vi "acquireWhenClick.vi"() -> ()   [LabVIEW 2016]
uses:
  <vilib>/Utility/file.llb/Write Delimited Spreadsheet (DBL).vi
panel:
  out "即将记录":dbl=1.0
  out "osc stoped":bool
  in  "OSC in":refnum<visa-resource-name>
  in  "start":bool
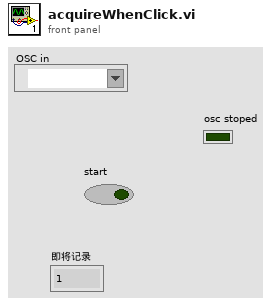
[diagram p1: front panel]
types:
  T1 = typedef "NI_Matrix.lvlib/RealMatrix.ctl" = dbl[][]
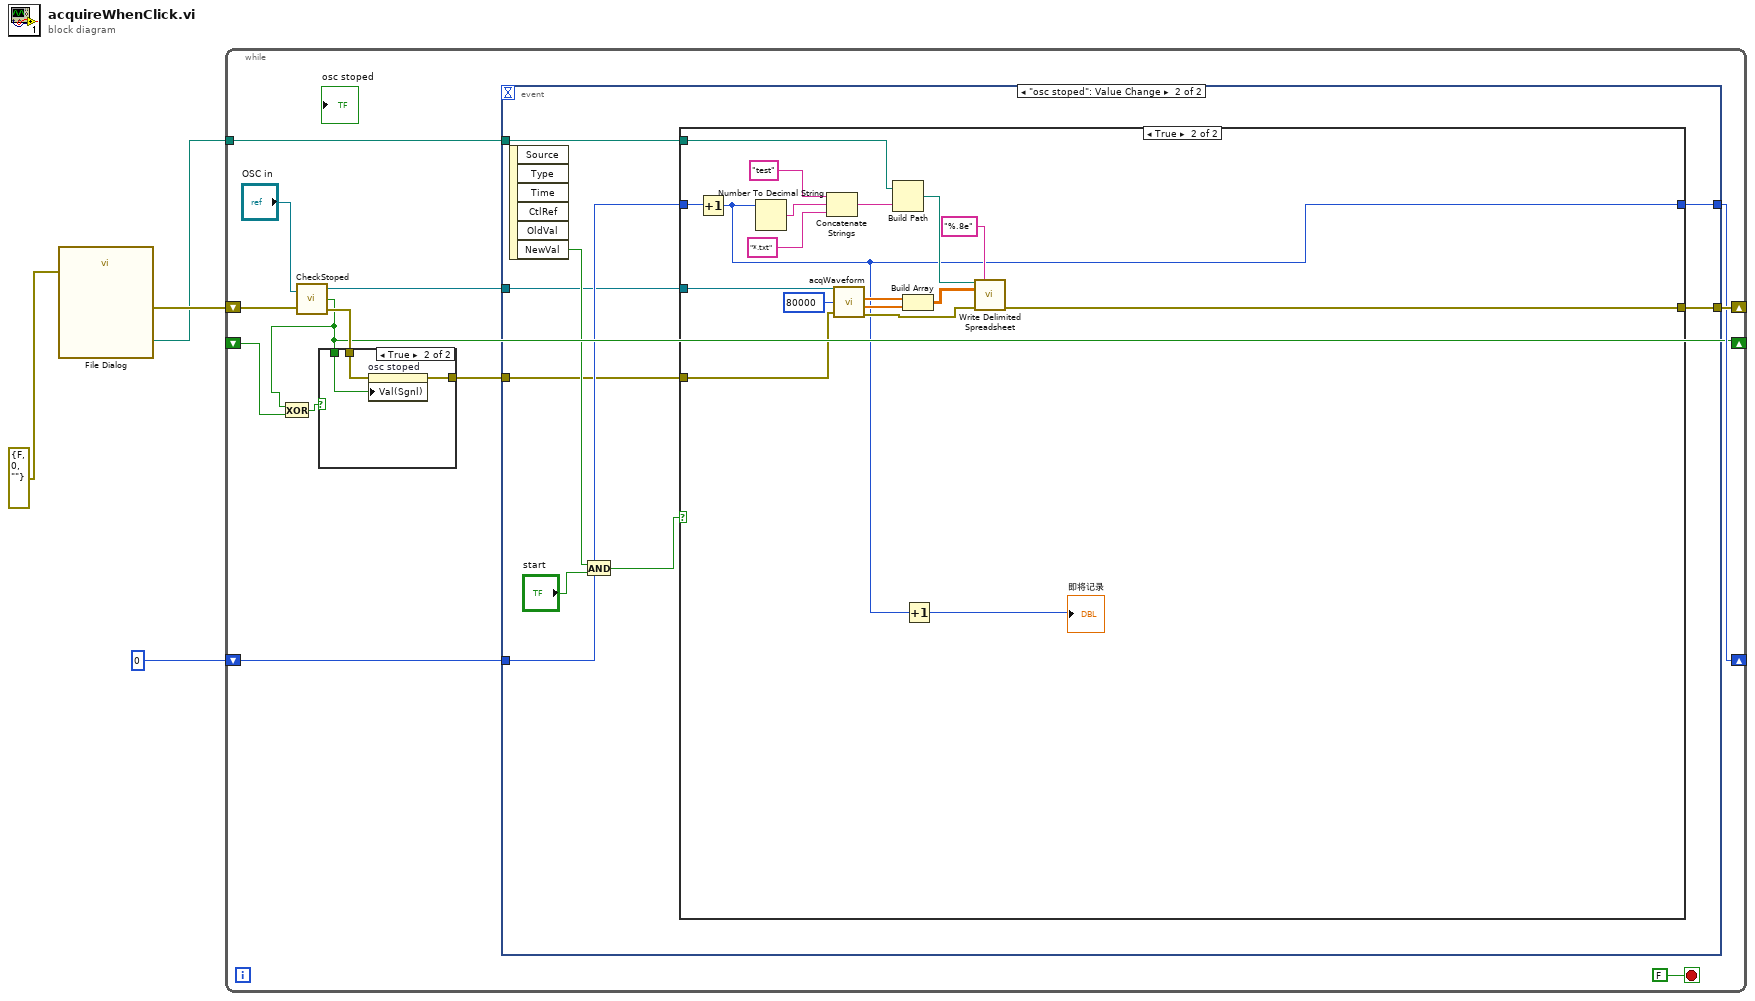
[diagram p0: block diagram]
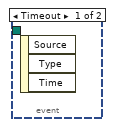
[diagram p3: hidden frame]
diagram:
  n1 = call "File Dialog"("error in"=errorcluster {"status"=FALSE, "code"=0, "source"=""} ("error in (no error)")) -> ("selected path"=w1:path, "error out"=w2:errorcluster)  [unwired: 11 in, 2 out]
  n2 = while {
    tunnel: w1 -> [w10]
    shift-right: [w9] -> _
    shift-left: w2 -> [w16]
    shift-right: [w8] -> _
    shift-left: 0 -> [w13]
    shift-right: [w6] -> _
    shift-left: _ -> [w7]
    stop <- FALSE stop-if-true
    n3 = call "CheckStoped.vi"("OSC in"="OSC in", "error in (no error)"=w16) -> ("OSC out"=w12:refnum<visa-resource-name>, "Stopped?"=w6:bool, "error out"=w14:errorcluster)
    n4 = Exclusive Or(1:w7, 2:w6) -> (0:w5:bool)
    n5 = case shown="True" w5 {
      tunnel: w14 -> [w18 w21]
      tunnel: [w18 w20] -> w11
      tunnel: w6 -> [_ w19]
      frame False {
      }
      frame True {
        n6 = property on="osc stoped" class="Bool (strict)"(error in=w21, "Val(Sgnl)"=w19) -> (error out=w20:errorcluster)  [unwired: 1 in, 1 out]
      }
    }
    n7 = event shown="[1] \"osc stoped\": Value Change" {
      selector: _ -> [_ _]
      dyn-events: _ -> [_ _]
      timeout: _ -> [_ _]
      tunnel: w13 -> [_ w27]
      tunnel: w12 -> [_ w26]
      tunnel: w11 -> [_ w25]
      tunnel: w10 -> [_ w24]
      tunnel: [_ w23] -> w9
      tunnel: [_ w22] -> w8
      event Timeout {
        n8 = event-data() -> ()  [unwired: 1 in, 3 out]
      }
      event "osc stoped": Value Change {
        n9 = event-data() -> ("NewVal"=w29:bool)  [unwired: 1 in, 5 out]
        n10 = And(x=w29, y="start") -> (x .and. y?=w28:bool)
        n11 = case shown="True" w28 {
          tunnel: w27 -> [w31 w50]
          tunnel: w26 -> [_ w49]
          tunnel: w25 -> [w32 w47]
          tunnel: w24 -> [_ w39]
          tunnel: [w32 w35] -> w23
          tunnel: [w31 w33] -> w22
          frame False {
          }
          frame True {
            n12 = Increment(x=w50) -> (x+1=w33:i32)
            n13 = Number To Decimal String(number=w33) -> (decimal integer string=w43:string)  [unwired: 1 in]
            n14 = Concatenate Strings("test" ("string"), w43, "*.txt" ("string")) -> (w40:string)
            n15 = call "acqWaveform.vi"("OSC in"=w49, "Points"=u32 80000, "error in (no error)"=w47) -> ("time sequence"=w46:dbl[], "Voltage sequence"=w45:dbl[], "error out"=w36:errorcluster)  [unwired: 1 out]
            n16 = Build Path(base path=w39, name or relative path=w40) -> (appended path=w38:path)
            n17 = Build Array(w46, w45) -> (w44:T1)
            n18 = Increment(x=w33) -> (x+1=→"即将记录":i32)
            n19 = call-poly <vilib>:"Write Delimited Spreadsheet.vi"("file path (dialog if empty)"=w38, "format (%.3f)"="%.8e", "2D data"=w44, "error in (no error)"=w36) -> ("error out"=w35:errorcluster)  [unwired: 10 in, 1 out]
          }
        }
      }
    }
  }
